vi "Connect.vi"(8 "Error In":errorcluster, 10 "Resource Name":refnum<k15>, 11 "object in":refnum<class "Disconnected.lvclass">) -> (0 "Error Out":errorcluster, 2 "Resource Name out":refnum<k15>, 3 ":FGEN State":refnum<class "IStates.lvclass">)   [LabVIEW 2023, in "HAL.lvlib" / "PXI-5441.lvlib" / "Disconnected.lvclass"]
uses:
  Disconnected.lvclass
  IFGEN_interface/IStates_interface/IStates.lvclass
  Connected_class/Connected.lvclass
  Error_class/Error.lvclass
  Disconnected.lvclass/Disconnected.ctl
  D:/git/HAL/PXI-5441_class/states/Connected_class/Connected.lvclass
  D:/git/HAL/IFGEN_interface/IStates_interface/IStates.lvclass
  D:/git/HAL/PXI-5441_class/states/Error_class/Error.lvclass
  D:/git/HAL/PXI-5441_class/states/Disconnected_class/Disconnected.lvclass
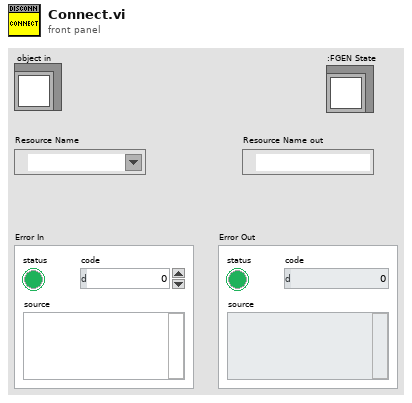
[diagram p1: front panel]
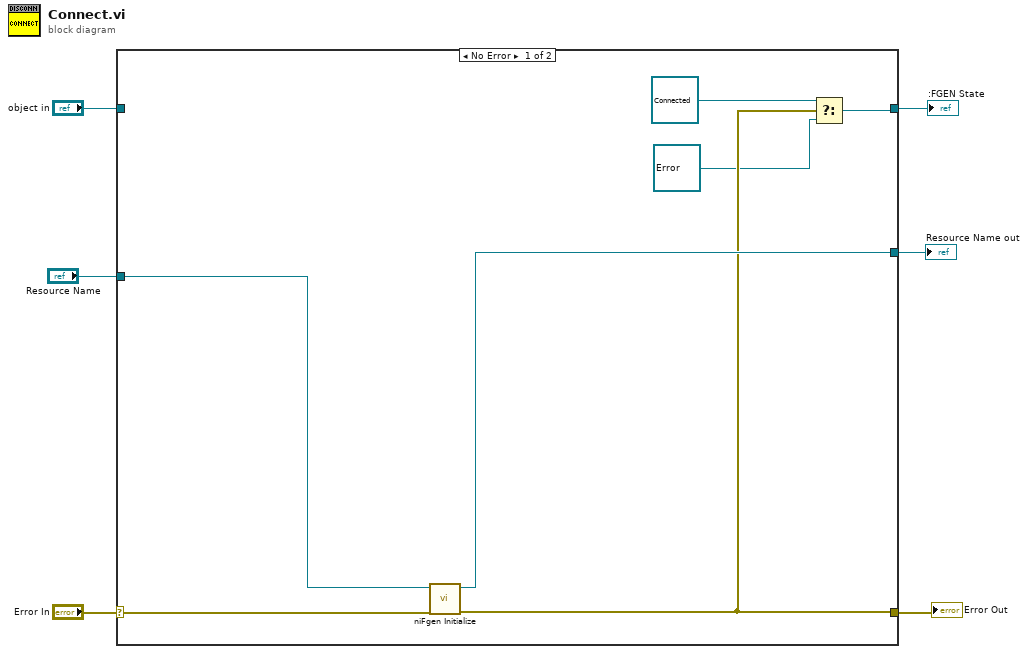
[diagram p0: block diagram]
diagram:
  n1 = case shown="No Error" "Error In" {
    selector: "Error In" -> [w13 w16]
    tunnel: [w10 w16] -> w5
    tunnel: [w7 w15] -> w1
    tunnel: "object in" -> [_ w15]
    tunnel: "Resource Name" -> [w12 w14]
    tunnel: [w11 w14] -> w2
    frame No Error {
      n2 = call <instrlib>:"niFgen Initialize.vi"("error in (no error)"=w13, "Resource Name"=w12) -> ("error out"=w10:errorcluster, "Instrument Handle Out"=w11:refnum<k15>)  [unwired: 8 in]
      n3 = Select(t=refnum<class "Connected.lvclass"> refnum ("PXI-5441.lvlib:Connected"), s=w10, f=refnum<class "Error.lvclass"> refnum ("PXI-5441.lvlib:Error")) -> (s? t:f=w7:refnum<class "IStates.lvclass">)
    }
    frame Error {
    }
  }
  "Error Out" <- w5
  "Resource Name out" <- w2
  ":FGEN State" <- w1
